vi "Test LRS Methods.vi"() -> ()   [LabVIEW 2014]
uses:
  <vilib>/Analysis/Matrix/Datatypes/RealMatrix.ctl
  <vilib>/Analysis/baseanly.llb/Real Determinant.vi
  <vilib>/Analysis/7linalg.llb/Solve Linear Equations (single right hand).vi
  <vilib>/Analysis/baseanly.llb/Solve Linear Equations By Cholesky.vi
  <vilib>/Analysis/baseanly.llb/Real Matrix to Compact Array.vi
  <vilib>/Analysis/baseanly.llb/Real Compact Tri-Matrix Linear Eqs.vi
  <vilib>/Analysis/1siggen.llb/Ramp Pattern by Delta.vi
  <vilib>/Analysis/Matrix/Numeric/Conversions/Array To Matrix - RA2.vi
  <vilib>/Analysis/baseanly.llb/Real Inverse Matrix.vi
  <vilib>/Analysis/7linalg.llb/Solve Linear Eqs (General).vi
  <vilib>/Analysis/7linalg.llb/Solve Linear Eqs (Gen, single right hand).vi
  Reusable/General/Math Utilities.lvlib
  <vilib>/Analysis/NI_AALBase.lvlib
  <vilib>/Analysis/Matrix/NI_Matrix.lvlib
  <vilib>/Analysis/NI_AALPro.lvlib
panel:
  out "cofactor":i64[](array[numeric]) format="%.3e"
  out "A":i64[](array[numeric]) format="%.2e"
  out "det(A)":i64 format="%.2e"
  out "determinant":dbl format="%.2e"
  out "error":i32
  out "Inverse":dbl[](array[numeric])
  out "Inverse Matrix":T1
  out "x/y 3":dbl[](array[numeric])
  out "Solution Vector":dbl[](array[numeric]) format="%.2f"
  out "Real Matrix":T1 format="%#.6f"
  in  "tau":dbl=65.0 format="%#_13g"
  in  "B":dbl format="%#_13g"
  in  "A":dbl=1.0 format="%#_13g"
  in  "stop":bool
  in  "end":dbl=1856.0 format="%#_13g"
  out "Waveform Graph":i64[](graph)
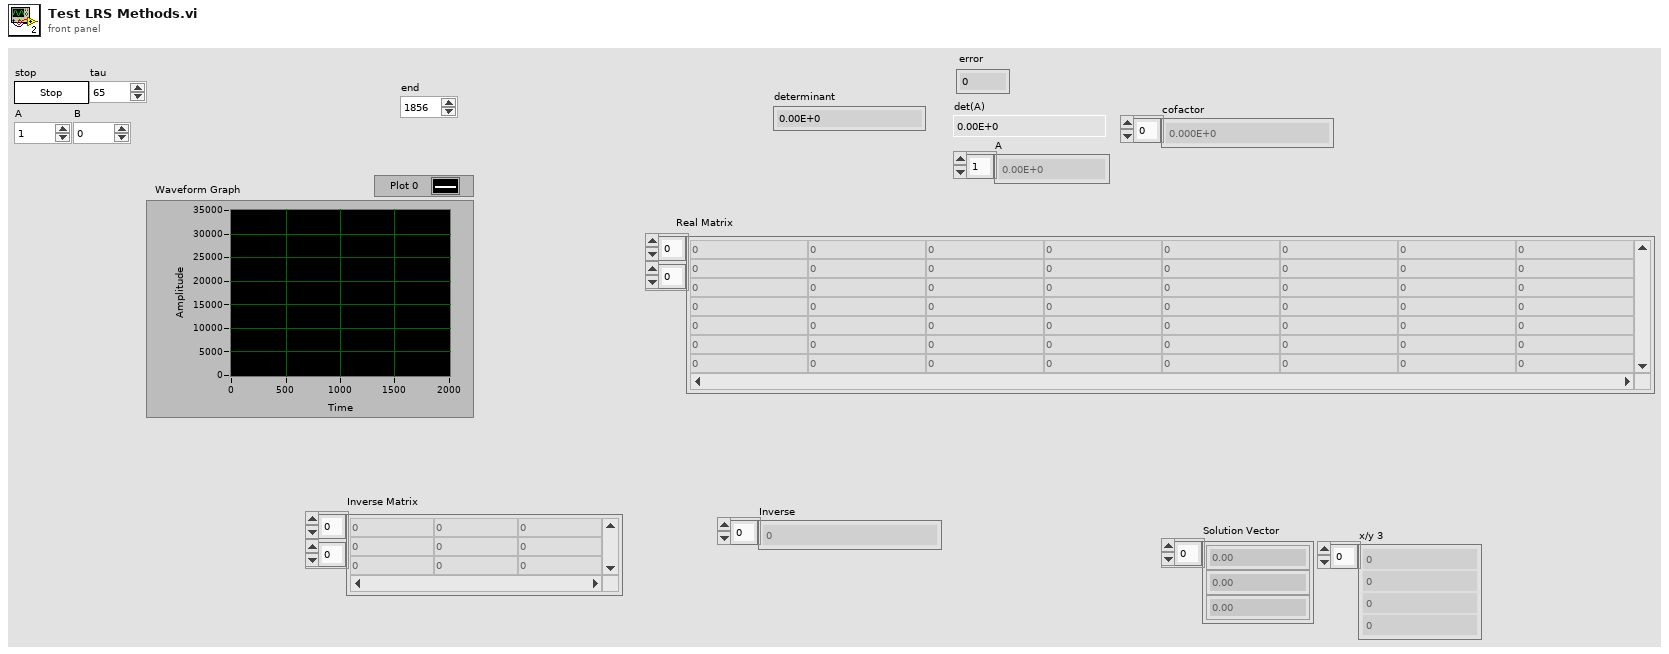
[diagram p1: front panel]
types:
  T1 = typedef "NI_Matrix.lvlib/RealMatrix.ctl" = dbl[][]
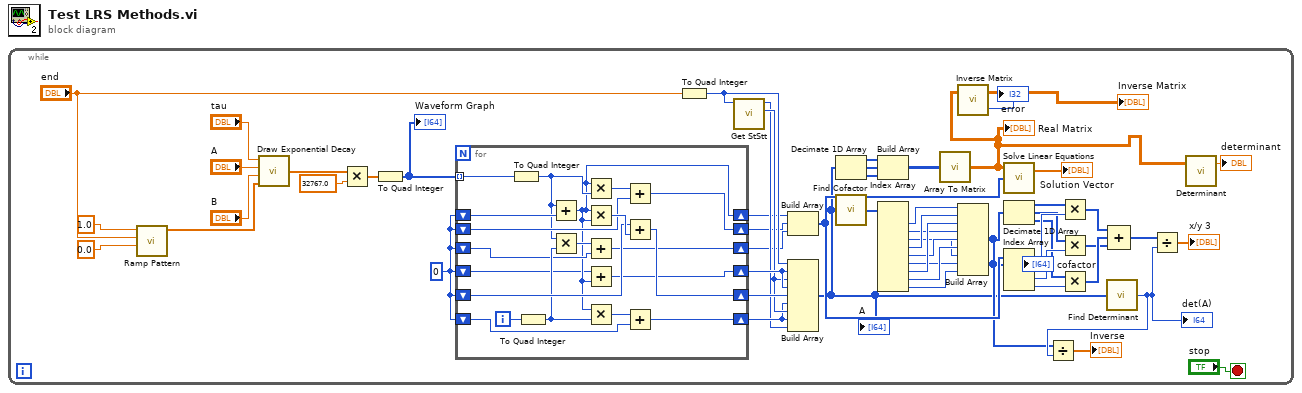
[diagram p0: block diagram]
diagram:
  n1 = while {
    stop <- "stop" stop-if-true
    w47 = i64 0
    n2 = call-poly <vilib>:"Ramp Pattern.vi"("start"=0.0, "end"="end", "delta"=1.0) -> ("Ramp Pattern"=w54:dbl[])  [unwired: 6 in, 2 out]
    n3 = call "Draw Exponential Decay.vi"("time"=w54, "B"="B", "A"="A", "tau"="tau") -> ("ExponentialOut"=w51:dbl[])
    n4 = Multiply(x=w51, y=32767.0) -> (x*y=w49:dbl[])
    n5 = To Quad Integer(1:w49) -> (0:w48:i64[])
    "Waveform Graph" <- w48
    n6 = for {
      shift-right: [w60] -> w32
      shift-left: w47 -> [w77]
      shift-right: [w74] -> w42
      shift-left: w47 -> [w75]
      shift-right: [w70] -> w40
      shift-left: w47 -> [w71]
      shift-right: [w69] -> w34
      shift-left: w47 -> [w67]
      shift-right: [w63] -> w33
      shift-left: w47 -> [w62]
      tunnel: w48 -> [w61] mode=indexing
      shift-right: [w59] -> w43
      shift-left: w47 -> [w58]
      i -> [w73]
      n7 = To Quad Integer(1:w61) -> (0:w66:i64)
      n8 = To Quad Integer(1:w73) -> (0:w65:i64)
      n9 = Add(x=w66, y=w77) -> (x+y=w60:i64)
      n10 = Multiply(x=w66, y=w65) -> (x*y=w64:i64)
      n11 = Multiply(x=w60, y=w66) -> (x*y=w68:i64)
      n12 = Multiply(x=w60, y=w60) -> (x*y=w76:i64)
      n13 = Add(x=w64, y=w62) -> (x+y=w63:i64)
      n14 = Add(x=w58, y=w60) -> (x+y=w59:i64)
      n15 = Multiply(x=w60, y=w65) -> (x*y=w72:i64)
      n16 = Add(x=w68, y=w67) -> (x+y=w69:i64)
      n17 = Add(x=w75, y=w76) -> (x+y=w74:i64)
      n18 = Add(x=w72, y=w71) -> (x+y=w70:i64)
    }
    n19 = To Quad Integer(1:"end") -> (0:w44:i64)
    n20 = call "Get StStt.vi"("N"=w44) -> ("St"=w41:u32, "Stt"=w39:u32)  [unwired: 9 in]
    n21 = Build Array(w32, w34, w33) -> (w11:i64[])
    n22 = Build Array(w44, w43, w41, w43, w42, w40, w41, w40, w39) -> (w3:i64[])
    "A" <- w3
    n23 = Decimate 1D Array(w3) -> (w38:i64[], w37:i64[], w36:i64[])
    n24 = call "Find Cofactor.vi"("A"=w3) -> ("cofA"=w30:i64[])  [unwired: 4 in]
    n25 = Build Array(w38, w37, w36) -> (w35:i64[][])
    n26 = Index Array(array=w30) -> (element #1=w29:i64, element #2=w26:i64, element #3=w23:i64, element #4=w28:i64, element #5=w25:i64, element #6=w22:i64, element #7=w27:i64, element #8=w24:i64, element #9=w21:i64)  [unwired: 9 in]
    n27 = call-poly <vilib>:"Array To Matrix.vi"("Real 2D Array"=w35) -> ("Real Matrix"=w1:T1)
    "Real Matrix" <- w1
    n28 = call-poly <vilib>:"Inverse Matrix.vi"("Input Matrix"=w1) -> ("error"=→"error":i32, "Inverse Matrix"=→"Inverse Matrix":T1)  [unwired: 1 in]
    n29 = Build Array(w29, w28, w27, w26, w25, w24, w23, w22, w21) -> (w6:i64[])
    "cofactor" <- w6
    n30 = call-poly <vilib>:"Solve Linear Equations.vi"("Known Vector"=w11, "Input Matrix"=w1) -> ("Solution Vector"=→"Solution Vector":dbl[])  [unwired: 1 in, 1 out]
    n31 = Decimate 1D Array(w6) -> (w20:i64[], w18:i64[], w16:i64[])
    n32 = Index Array(array=w11) -> (element #1=w19:i64, element #2=w17:i64, element #3=w15:i64)  [unwired: 3 in]
    n33 = Multiply(x=w20, y=w19) -> (x*y=w14:i64[])
    n34 = Multiply(x=w18, y=w17) -> (x*y=w12:i64[])
    n35 = Multiply(x=w16, y=w15) -> (x*y=w13:i64[])
    n36 = call "Find Determinant.vi"("A"=w3) -> ("det(A)"=w7:i64)  [unwired: 4 in]
    "det(A)" <- w7
    n37 = Divide(x=w6, y=w7) -> (x/y=→"Inverse":dbl[])
    n38 = Compound Arithmetic op=ADD(w14, w13, w12) -> (w10:i64[])
    n39 = Divide(x=w10, y=w7) -> (x/y=→"x/y 3":dbl[])
    n40 = call-poly <vilib>:"Determinant.vi"("Input Matrix"=w1) -> ("determinant"=→"determinant":dbl)  [unwired: 1 in, 1 out]
  }
